vi "FTW-Actor-AddJob-Next.vi"(1 "Add Next in Job Queue":string, 3 "FTW Actor Instance":refnum<class "FTW-ActorInstance.lvclass">) -> (0 "FTW Actor Instance out":refnum<class "FTW-ActorInstance.lvclass">)   [LabVIEW 2012, in "FTW-Actor.lvlib" / "FTW-ActorInstance.lvclass"]
uses:
  FTW-ActorInstance.lvclass
  FTW-ActorInstance.lvclass/FTW-ActorInstance.ctl
  JobSequencer/FTW-JobSequencer.lvclass/FTW-JobSequencer.ctl
  JobSequencer/FTW-JobSequencer.lvclass
panel:
  # "Inputs"
  # "Outputs"
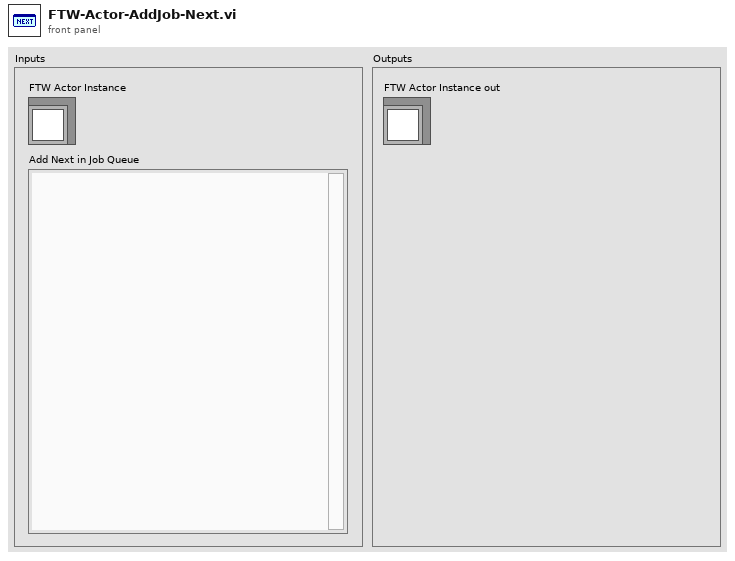
[diagram p1: front panel]
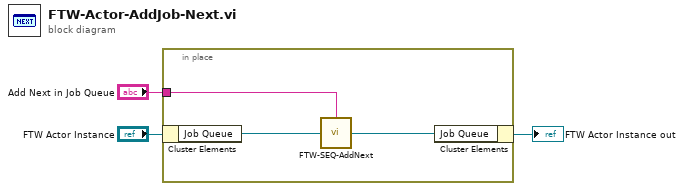
[diagram p0: block diagram]
diagram:
  n1 = in-place {
    in-place-border: "Add Next in Job Queue" -> [w4]
    n2 = in-place-cluster #1("FTW Actor Instance") -> ("Job Queue"=w6:refnum<class "FTW-JobSequencer.lvclass">)
    n3 = call "FTW-SEQ-AddNext.vi"("Add Next in Sequence"=w4, "Sequencer"=w6) -> ("Sequencer out"=w5:refnum<class "FTW-JobSequencer.lvclass">)  [unwired: 2 in]
    n4 = in-place-cluster #1("Job Queue"=w5) -> (→"FTW Actor Instance out":refnum<class "FTW-ActorInstance.lvclass">)
  }
